vi "题目5.vi"() -> ()   [LabVIEW 2017]
panel:
  out "通过":bool
  out "你没有通过考试！":bool
  out "恭喜":bool
  in  "数值":dbl
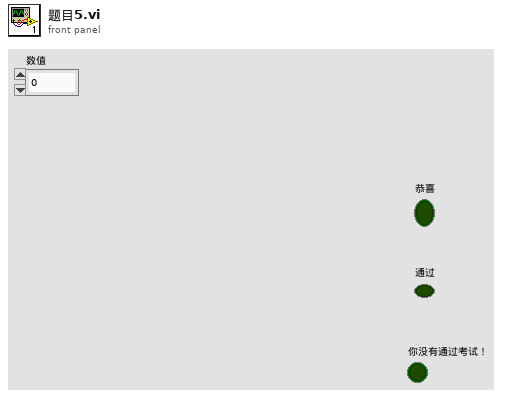
[diagram p1: front panel]
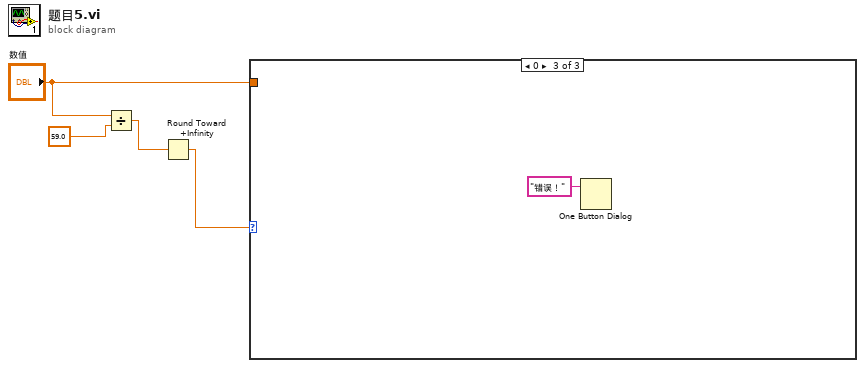
[diagram p0: block diagram]
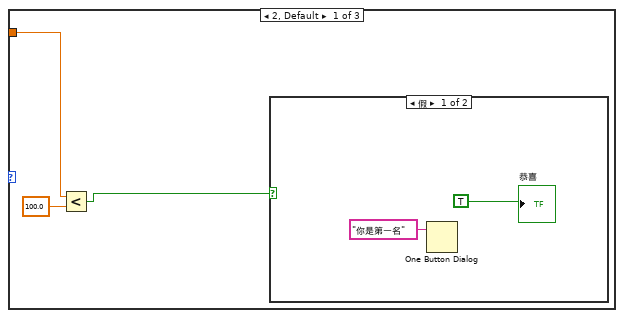
[diagram p2: hidden frame]
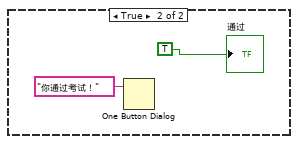
[diagram p3: hidden frame]
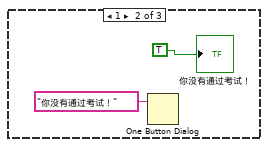
[diagram p4: hidden frame]
diagram:
  n1 = Divide(x="数值", y=59.0) -> (x/y=w2:dbl)
  n2 = Round Toward +Infinity(x=w2) -> (ceil(x): smallest int >= x=w1:dbl)
  n3 = case shown="0" w1 {
    tunnel: "数值" -> [w5 _ _]
    frame 2, Default {
      n4 = Less?(x=w5, y=100.0) -> (x < y?=w6:bool)
      n5 = case shown="假" w6 {
        frame False {
          n6 = One Button Dialog(message="你是第一名" ("消息")) -> ()  [unwired: 1 in, 1 out]
          "恭喜" <- TRUE
        }
        frame True {
          n7 = One Button Dialog(message="你通过考试！" ("消息")) -> ()  [unwired: 1 in, 1 out]
          "通过" <- TRUE
        }
      }
    }
    frame 1 {
      n8 = One Button Dialog(message="你没有通过考试！" ("消息")) -> ()  [unwired: 1 in, 1 out]
      "你没有通过考试！" <- TRUE
    }
    frame 0 {
      n9 = One Button Dialog(message="错误！" ("消息")) -> ()  [unwired: 1 in, 1 out]
    }
  }
